vi "Write Binary Config.vi"(4 "Include Class Name":bool, 6 "byte order (0:big-endian, network order)":T1(ring), 8 "error in (no error)":errorcluster, 11 "Subset_STR in":refnum<class "Insert_STR.lvclass">) -> (0 "error out":errorcluster, 2 "Binary":string, 3 "Subset_STR out":refnum<class "Insert_STR.lvclass">)   [LabVIEW 2021, in "Insert_STR.lvclass"]
uses:
  Insert_STR.lvclass
  Insert_STR.lvclass/Insert_STR.ctl
  Abs_Types/String/Abs_String.lvclass
  Abs_Types/Numeric/Abs_Numeric.lvclass
  Abs_Types/Value/Abs_Value.lvclass
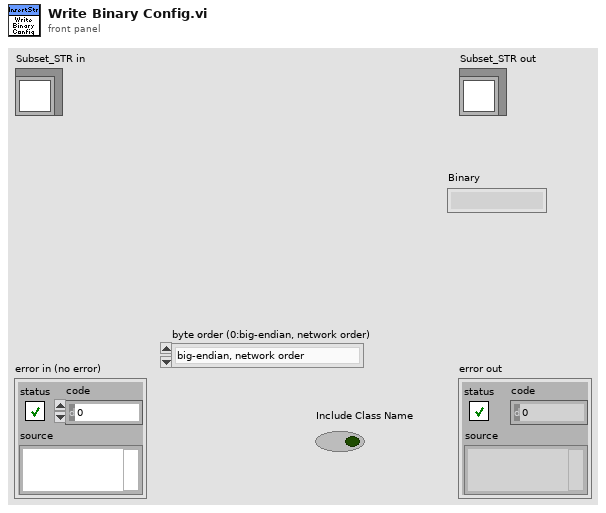
[diagram p1: front panel]
types:
  T1 = enum16{"big-endian, network order", "native, host order", "little-endian"}
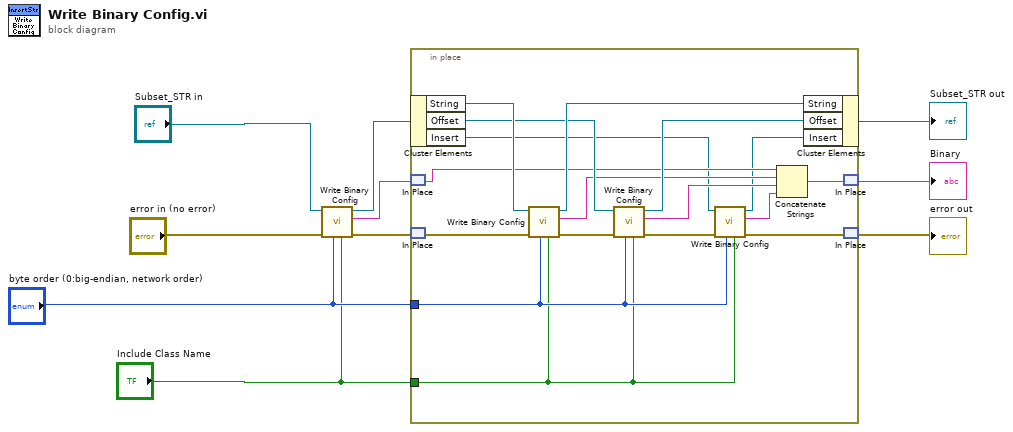
[diagram p0: block diagram]
diagram:
  n1 = call-parent "Write Binary Config.vi"("Include Class Name"="Include Class Name", "byte order (0:big-endian, network order)"="byte order (0:big-endian, network order)", "error in (no error)"="error in (no error)", "Abs_Type in"="Subset_STR in") -> ("error out"=w2:errorcluster, "Binary"=w1:string, "Abs_Type out"=w3:refnum<class "Insert_STR.lvclass">)  [unwired: 5 in]
  n2 = in-place {
    in-place-border: "byte order (0:big-endian, network order)" -> [w12]
    in-place-border: "Include Class Name" -> [w11]
    n3 = in-place-cluster #1(w3) -> ("String"=w25:refnum<class "Abs_String.lvclass">, "Offset"=w24:refnum<class "Abs_Numeric.lvclass">, "Insert"=w15:refnum<class "Abs_Value.lvclass">)
    n4 = in-place-match #2(w1) -> (w20:string)
    n5 = in-place-match #3(w2) -> (w27:errorcluster)
    n6 = call-dynamic "Write Binary Config.vi"("Include Class Name"=w11, "byte order (0:big-endian, network order)"=w12, "error in (no error)"=w27, "Abs_Type in"=w25) -> ("error out"=w22:errorcluster, "Binary"=w19:string, "Abs_Type out"=w26:refnum<class "Abs_String.lvclass">)  [unwired: 5 in]
    n7 = call-dynamic "Write Binary Config.vi"("Include Class Name"=w11, "byte order (0:big-endian, network order)"=w12, "error in (no error)"=w22, "Abs_Type in"=w24) -> ("error out"=w17:errorcluster, "Binary"=w21:string, "Abs_Type out"=w23:refnum<class "Abs_Numeric.lvclass">)  [unwired: 5 in]
    n8 = call-dynamic "Write Binary Config.vi"("Include Class Name"=w11, "byte order (0:big-endian, network order)"=w12, "error in (no error)"=w17, "Abs_Type in"=w15) -> ("error out"=w16:errorcluster, "Binary"=w13:string, "Abs_Type out"=w14:refnum<class "Abs_Value.lvclass">)  [unwired: 5 in]
    n9 = Concatenate Strings(w20, w19, w21, w13) -> (w18:string)
    n10 = in-place-cluster #1("String"=w26, "Offset"=w23, "Insert"=w14) -> (→"Subset_STR out":refnum<class "Insert_STR.lvclass">)
    n11 = in-place-match #2(w18) -> (→"Binary":string)
    n12 = in-place-match #3(w16) -> (→"error out":errorcluster)
  }
